vi "UI_FocusList.vi"() -> ()   [LabVIEW 2016]
uses:
  <vilib>/Utility/error.llb/DialogType.ctl
  DAQ-Display/PanelSplitToolkit/QueueManager.llb/Insert.vi
  DAQ-Display/PanelSplitToolkit/QueueManager.llb/Remove.vi
  Controls/DAQListOperation.ctl
  DAQ-Display/PanelSplitToolkit/QueueManager.llb/Valid?.vi
  DAQ-Display/PanelSplitToolkit/QueueManager.llb/Destroy.vi
  DAQ-Display/PanelSplitToolkit/QueueManager.llb/CreatQueue.vi
panel:
  out "波形图表":waveform(dbl)[](graph)
  out "ItemTag":string
  in  "Caller":string
  out "DAQList":i32(listbox)
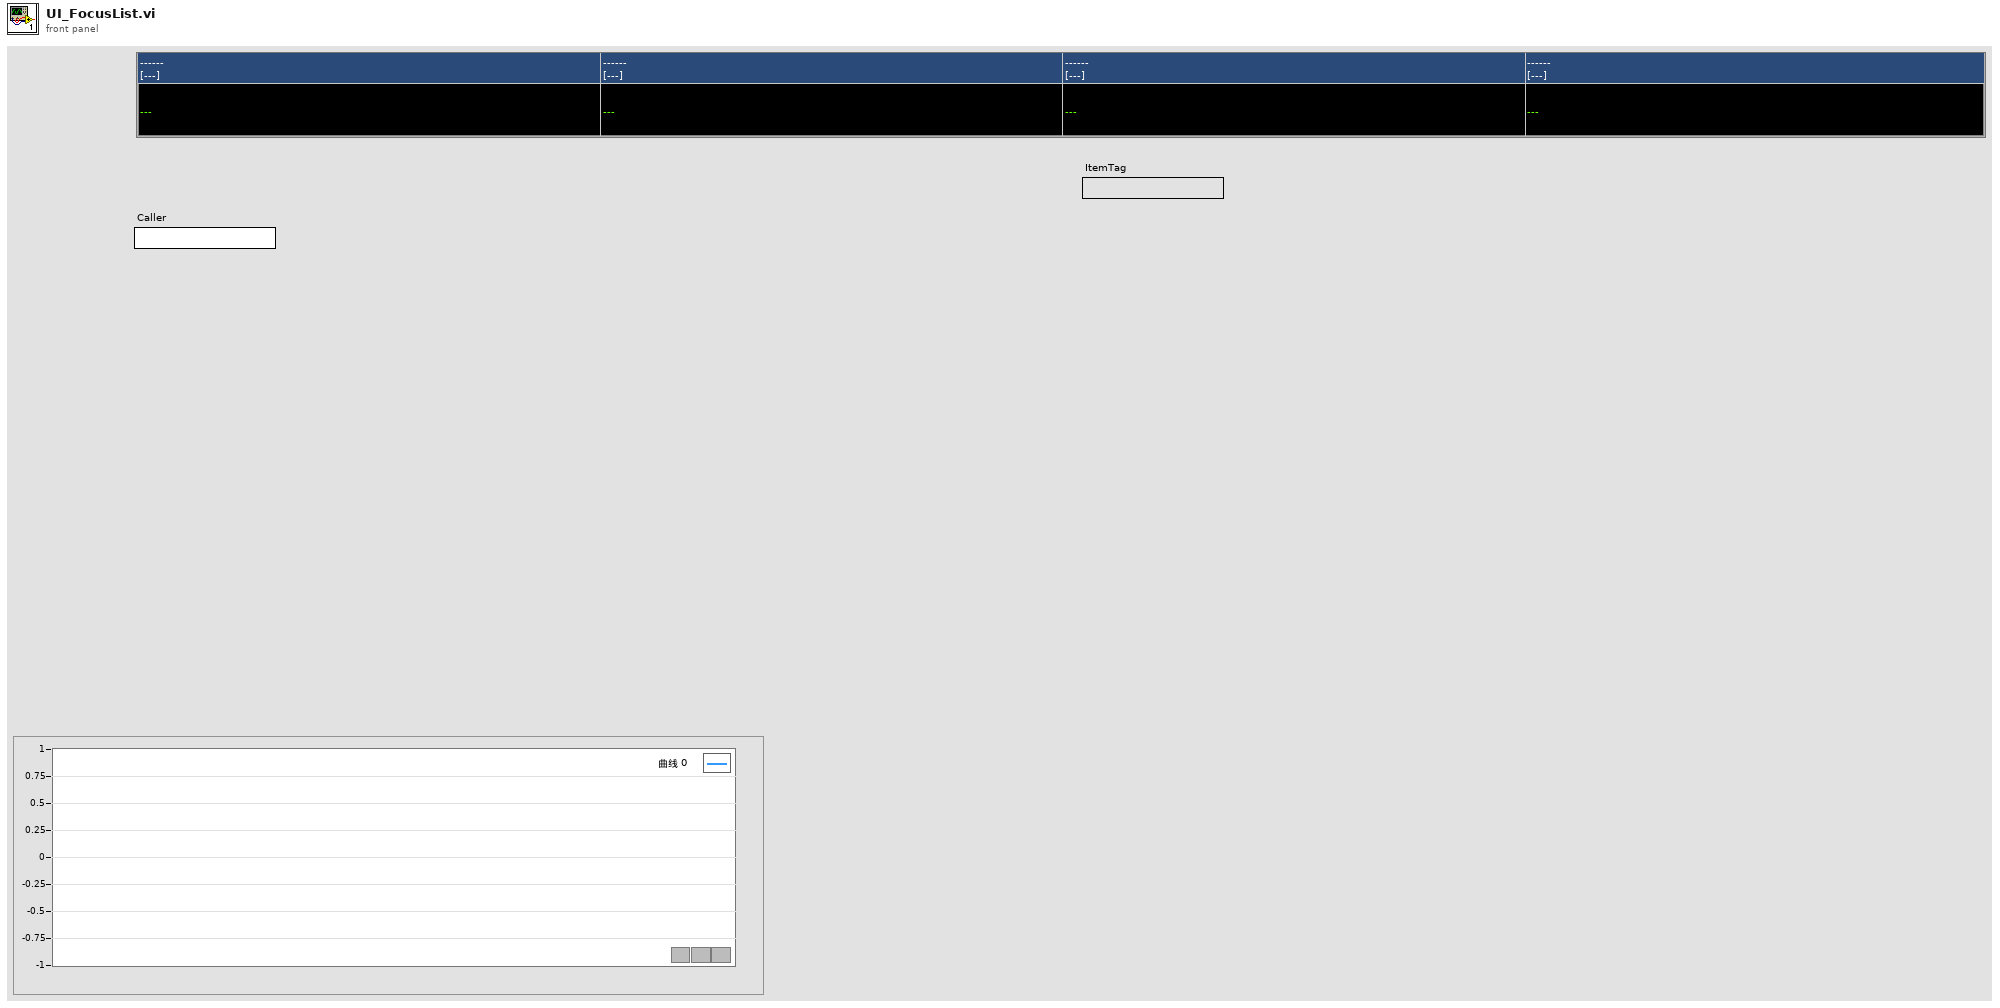
[diagram p1: front panel]
types:
  T1 = cluster{"error":errorcluster, "LocalQ":cluster{"LQName":string, "LQEvent":string, "LQData":variant}, "HighQ":cluster{"HQName":string, "HQEvent":string, "HQData":variant}}
  T2 = typedef "LVPoint32TypeDef.ctl" = cluster{"Horizontal":i32, "Vertical":i32}
  T3 = typedef "LVRowAndColumnTypeDef.ctl" = cluster{"Row":i32, "Column":i32}
  T4 = typedef "DAQListOperation.ctl" = enum16{"Init", "Clear", "Update Data", "Update CH Name", "Set List Property", "Get CHTag[]"}
  T5 = typedef "DialogType.ctl" = u16
  T6 = typedef "PCM PanelSplit.lvclass/Display Config.ctl" = cluster{"Display Mode":T7, "ChTag[]":string[], "window":T8, "Range":T9}
  T7 = typedef "PCM PanelSplit.lvclass/Display Mode.ctl" = enum16{"时域", "频谱", "功率谱"}
  T8 = typedef "NI_AALPro.lvlib/windowTd.ctl" = u32
  T9 = typedef "LVRangeTypeDef.ctl" = cluster{"Minimum":dbl, "Maximum":dbl, "Increment":dbl, "Minor Increment":dbl, "Start":dbl}
  T10 = cluster{"error":errorcluster, "LocalQ":cluster{"LQName":string, "LQEvent":string, "LQData":variant}, "HighQ":cluster{"HQName":string, "HQEvent":string, "HQData":variant}, "Display Config":T6, "波形图":refnum<vi>}
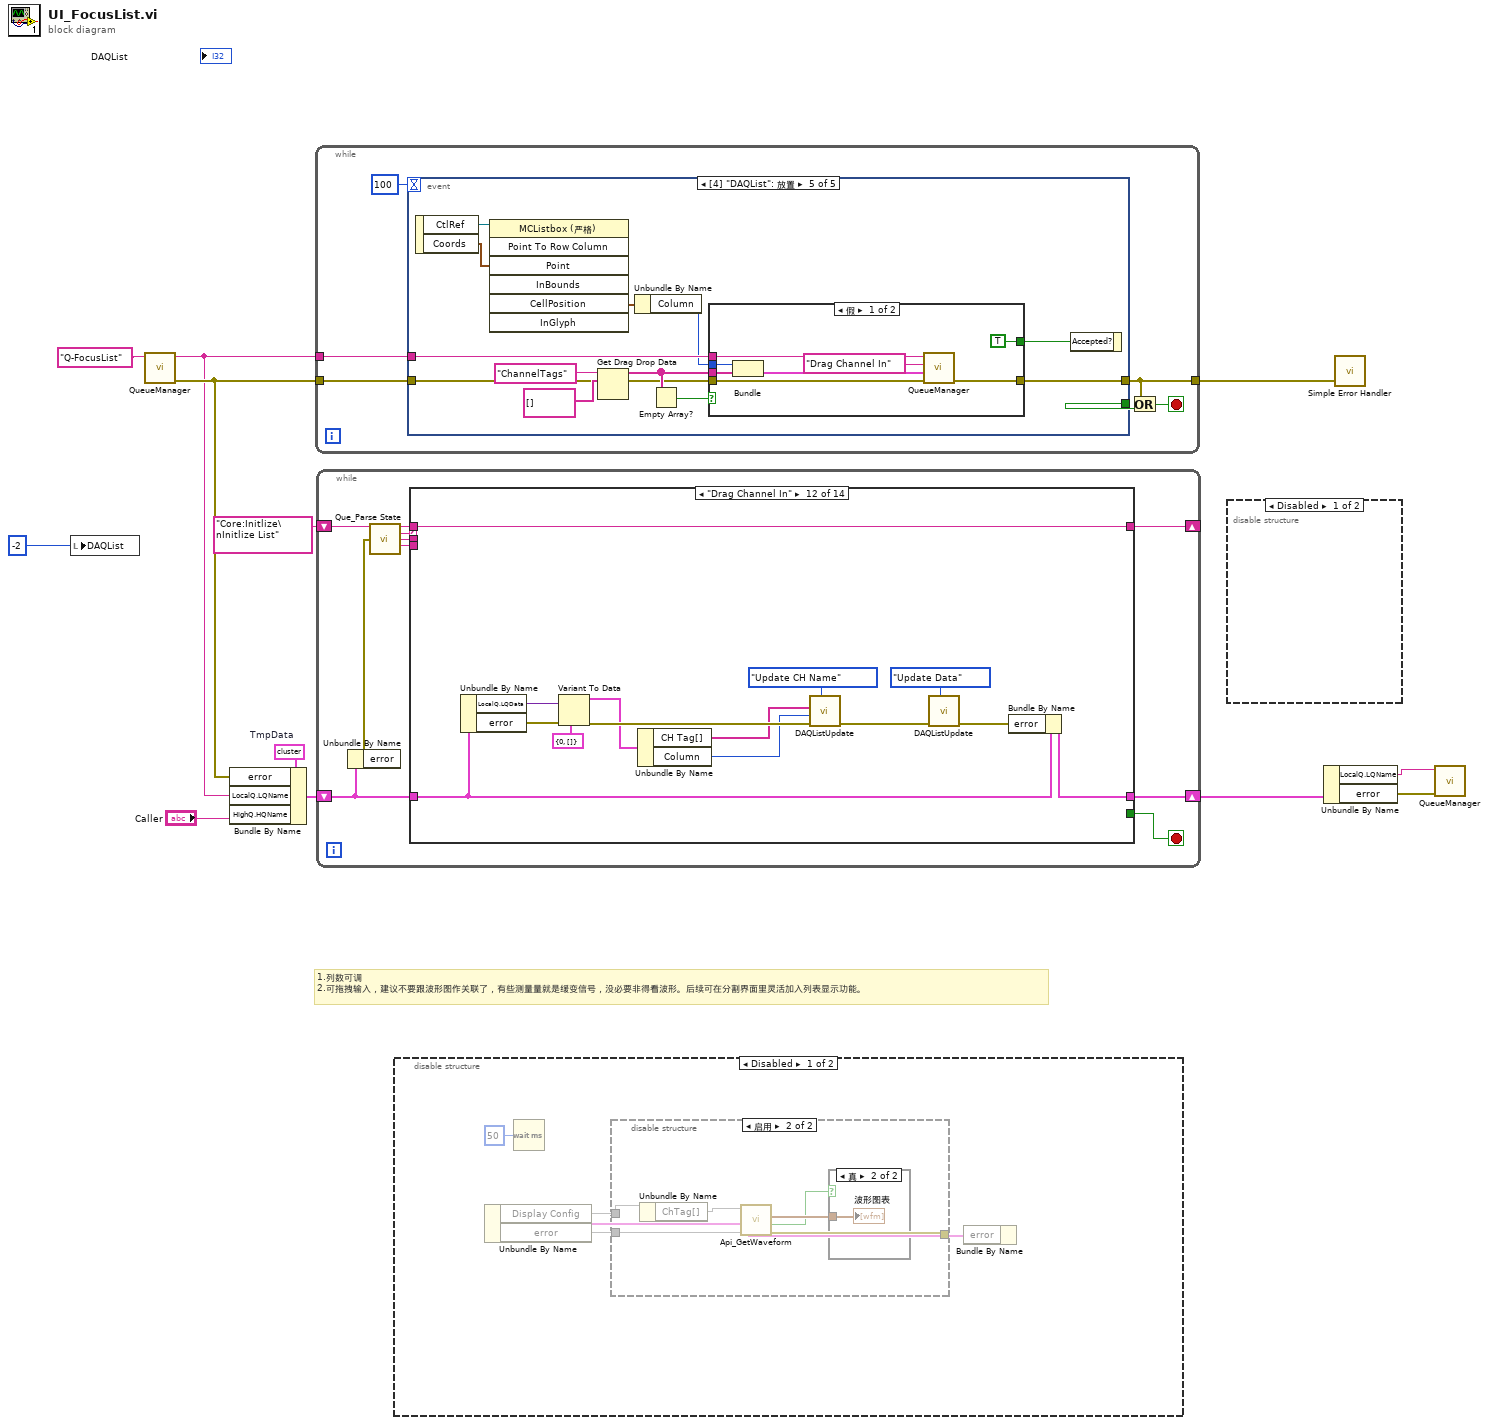
[diagram p0: block diagram]
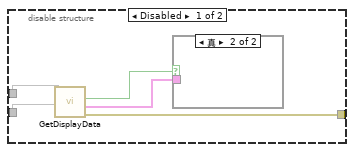
[diagram p2: hidden frame]
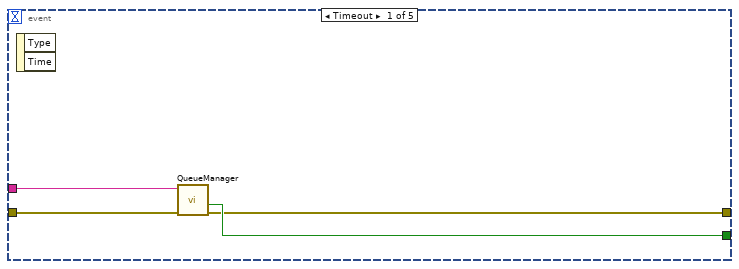
[diagram p7: hidden frame]
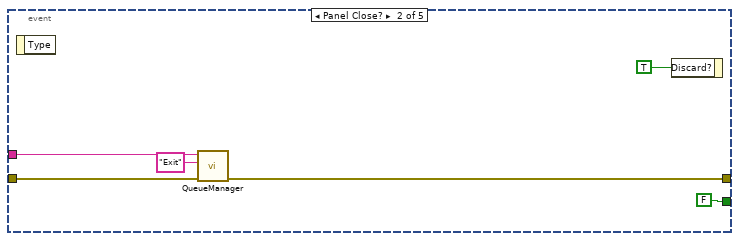
[diagram p8: hidden frame]
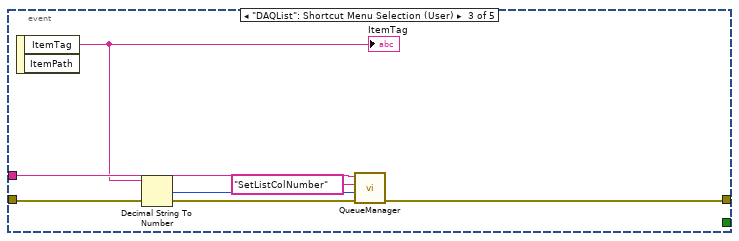
[diagram p9: hidden frame]
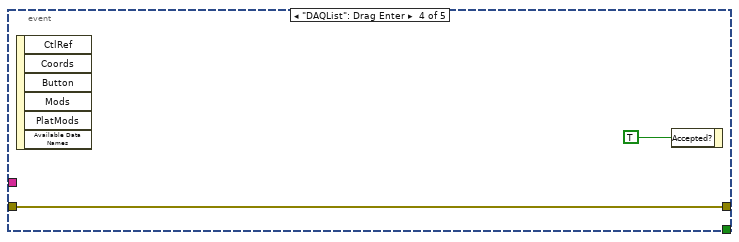
[diagram p10: hidden frame]
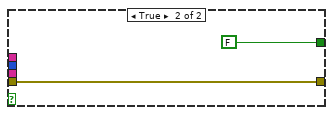
[diagram p11: hidden frame]
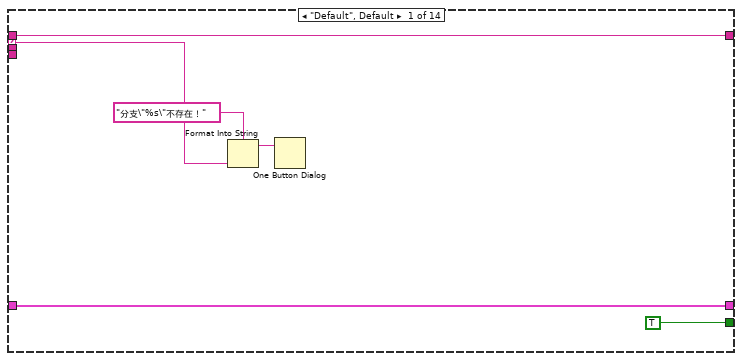
[diagram p12: hidden frame]
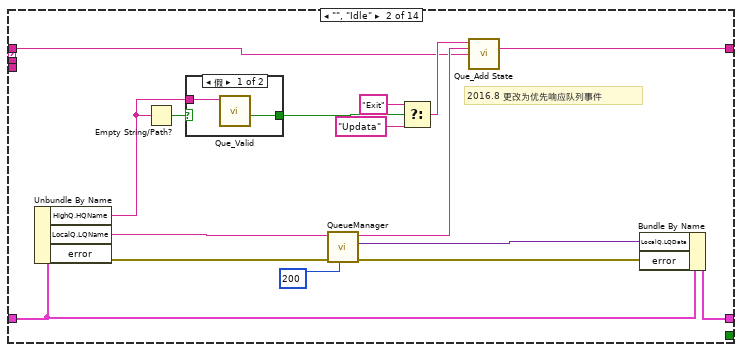
[diagram p13: hidden frame]
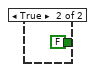
[diagram p14: hidden frame]
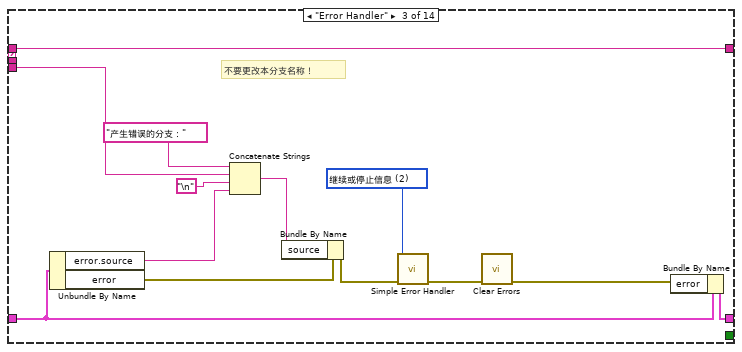
[diagram p15: hidden frame]
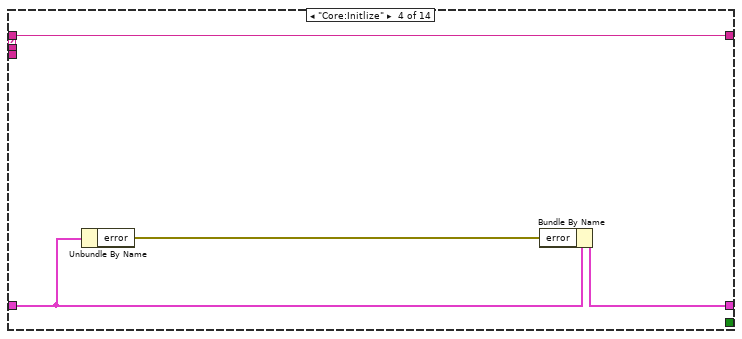
[diagram p16: hidden frame]
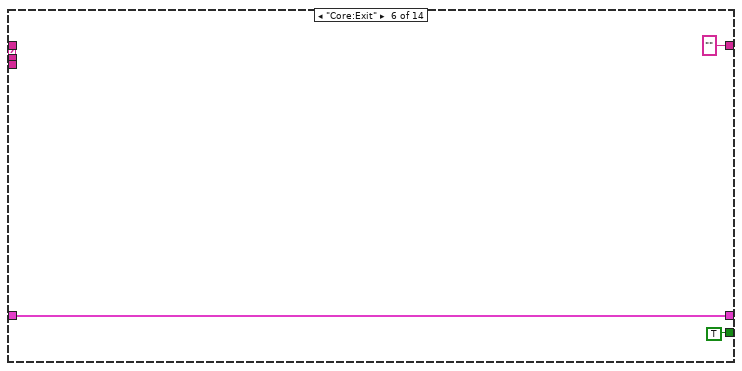
[diagram p18: hidden frame]
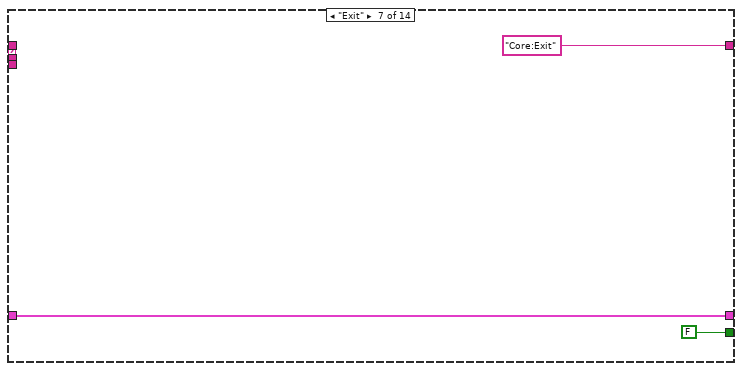
[diagram p19: hidden frame]
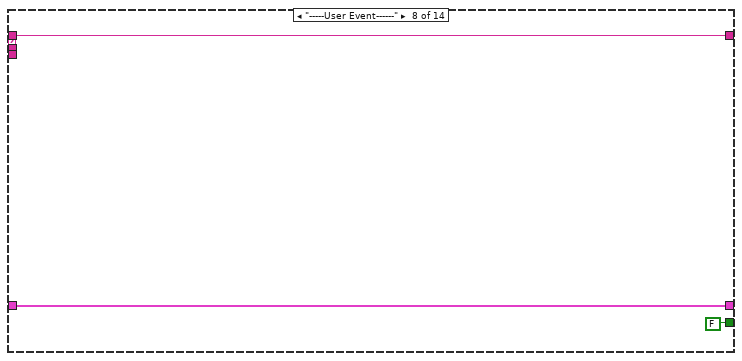
[diagram p20: hidden frame]
diagram:
  w8 = T1 {"error"={"status"=FALSE, "code"=0, "source"=""}, "LocalQ"={"LQName"="", "LQEvent"="", "LQData"=variant}, "HighQ"={"HQName"="", "HQEvent"="", "HQData"=variant}}  # TmpData
  # "1.列数可调\n2.可拖拽输入，建议不要跟波形图作关联了，有些测量量就是缓变信号，没必要非得看波形。后续可在分割界面里灵活加入列表显示功能。"
  n1 = local write "DAQList"(-2 ("Multicolumn Listbox")) -> ()
  n2 = call-poly "QueueManager.vi"("QueueName"="Q-FocusList") -> ("error out"=w4:errorcluster, "QueueName out"=w1:string)  [unwired: 9 in]
  n3 = Bundle By Name(cluster=w8, "error"=w4, "LocalQ.LQName"=w1, "HighQ.HQName"="Caller") -> (w7:T1)
  n4 = while {
    tunnel: w4 -> [w17]
    tunnel: w1 -> [w18]
    tunnel: [w14] -> w9
    stop <- w15 stop-if-true
    n5 = event shown="[4] \"DAQList\": 放置" {
      selector: _ -> [_ _ _ _ _]
      dyn-events: _ -> [_ _ _ _ _]
      timeout: 100 -> [_ _ _ _ _]
      tunnel: [w20 FALSE _ _ _] -> w16
      tunnel: w18 -> [w22 w27 w31 _ w43]
      tunnel: w17 -> [w21 w26 w33 w35 w44]
      tunnel: [w19 w25 w32 w35 w42] -> w14
      event Timeout {
        n6 = event-data() -> ()  [unwired: 1 in, 2 out]
        n7 = call-poly "QueueManager.vi"("error in (no error)"=w21, "Queue Name(unamed)"=w22) -> ("error out"=w19:errorcluster, "Not Exist?"=w20:bool)  [unwired: 8 in]
      }
      event Panel Close? {
        n8 = event-data() -> ()  [unwired: 1 in, 1 out]
        n9 = call-poly "QueueManager.vi"("error in"=w26, "Event"="Exit", "QueueName"=w27) -> ("error out"=w25:errorcluster)  [unwired: 7 in, 1 out]
        n10 = event-data("Discard?"=TRUE ("放弃？")) -> ()  [unwired: 1 in, 1 out]
      }
      event "DAQList": Shortcut Menu Selection (User) {
        n11 = event-data() -> ("ItemTag"=w30:string)  [unwired: 1 in, 1 out]
        "ItemTag" <- w30
        n12 = Decimal String To Number(string=w30) -> (number=w29:i32)  [unwired: 2 in, 1 out]
        n13 = call-poly "QueueManager.vi"("error in"=w33, "Data"=w29, "Event"="SetListColNumber", "QueueName"=w31) -> ("error out"=w32:errorcluster)  [unwired: 6 in, 1 out]
      }
      event "DAQList": Drag Enter {
        n14 = event-data() -> ()  [unwired: 1 in, 6 out]
        n15 = event-data("Accepted?"=TRUE) -> ()  [unwired: 1 in, 1 out]
      }
      event "DAQList": Drop {
        n16 = event-data() -> ("CtlRef"=w40:refnum<vi>, "Coords"=w39:T2)  [unwired: 1 in]
        n17 = invoke class="MCListbox (严格)" method="Point To Row Column"(reference=w40, "Point"=w39) -> ("CellPosition"=w38:T3)  [unwired: 5 in, 6 out]
        n18 = Get Drag Drop Data(8:string[] [], 9:"ChannelTags" ("数据名称")) -> (3:w47:string[])  [unwired: 1 in, 1 out]
        n19 = Unbundle By Name(w38) -> ("Column"=w37:i32)
        n20 = Empty Array?(array=w47) -> (empty?=w48:bool)
        n21 = case shown="假" w48 {
          tunnel: w44 -> [w56 w58]
          tunnel: [w55 w58] -> w42
          tunnel: w43 -> [w54 _]
          tunnel: w47 -> [w50 _]
          tunnel: [TRUE ("放弃？") FALSE ("放弃？")] -> w41
          tunnel: w37 -> [w51 _]
          frame False {
            n22 = Bundle("Column"=w51, w50) -> (w49:cluster{"Column":i32, string[]})  [unwired: 1 in]
            n23 = call-poly "QueueManager.vi"("error in"=w56, "Data"=w49, "Event"="Drag Channel In", "QueueName"=w54) -> ("error out"=w55:errorcluster)  [unwired: 6 in, 1 out]
          }
          frame True {
          }
        }
        n24 = event-data("Accepted?"=w41) -> ()  [unwired: 1 in, 1 out]
      }
    }
    n25 = Or(x=w14, y=w16) -> (x .or. y?=w15:bool)
  }
  n26 = while {
    shift-right: [w62] -> w10
    shift-left: w7 -> [w63]
    shift-right: [w61] -> _
    shift-left: "Core:Initlize\nInitlize List" -> [w68]
    stop <- w65 stop-if-true
    n27 = Unbundle By Name(w63) -> ("error"=w64:errorcluster)
    n28 = call "Que_Parse State.vi"("State Queue"=w68, "Error In (no error)"=w64) -> ("Remaining States"=w67:string, "Current State"=w66:string, "Arguments"=w60:string, "PreState"=w59:string)  [unwired: 10 in]
    n29 = case shown="\"Drag Channel In\"" w66 {
      selector: w66 -> [w72 _ _ _ _ _ _ _ _ _ _ _ _ _]
      tunnel: w67 -> [w73 w75 w106 w110 w112 _ _ w119 w128 w136 w150 w164 w178 w184]
      tunnel: w60 -> [_ _ _ _ _ _ _ _ _ _ _ _ _ _]
      tunnel: [TRUE _ _ _ _ TRUE FALSE FALSE _ _ _ _ _ _] -> w65
      tunnel: w63 -> [w74 w85 w103 w108 w111 w114 w117 w120 w124 w131 w149 w163 w177 w183]
      tunnel: [w74 w89 w102 w109 w111 w114 w117 w120 w122 w130 w143 w162 w176 w182] -> w62
      tunnel: [w73 w87 w106 w110 w112 "" ("Remaining States") "Core:Exit" ("Remaining States") w119 w128 w135 w150 w164 w178 w184] -> w61
      tunnel: w59 -> [_ _ w100 _ _ _ _ _ _ _ _ _ _ _]
      frame "Default", Default {
        n30 = Format Into String(format string="分支\"%s\"不存在！" ("格式字符串"), w72) -> (resulting string=w71:string)  [unwired: 2 in, 1 out]
        n31 = One Button Dialog(message=w71) -> ()  [unwired: 1 in, 1 out]
      }
      frame "", "Idle" {
        # "2016.8 更改为优先响应队列事件"
        n32 = Unbundle By Name(w85) -> ("HighQ.HQName"=w79:string, "LocalQ.LQName"=w84:string, "error"=w83:errorcluster)
        n33 = Empty String/Path?(string/path=w79) -> (empty?=w82:bool)
        n34 = case shown="假" w82 {
          tunnel: [w92 FALSE ("Not Exist?")] -> w81
          tunnel: w79 -> [w91 _]
          frame False {
            n35 = call "Que_Valid.vi"("Queue Name(unamed)"=w91) -> ("Not Exist?"=w92:bool)  [unwired: 9 in, 1 out]
          }
          frame True {
          }
        }
        n36 = call-poly "QueueManager.vi"("Time out(-1)"=200, "error in (no error)"=w83, "Queue Name"=w84) -> ("error out"=w90:errorcluster, "Data"=w88:variant, "Event"=w76:string)  [unwired: 5 in, 1 out]
        n37 = Select(t="Exit" ("Event"), s=w81, f="Updata") -> (s? t:f=w77:string)
        n38 = call "Que_Add State.vi"("State(s) in Front (\"\")"=w77, "State(s) in (\"\")"=w76, "State(s) at Back (\"\")"=w75) -> ("States Out"=w87:string)  [unwired: 12 in]
        n39 = Bundle By Name(cluster=w85, "LocalQ.LQData"=w88, "error"=w90) -> (w89:T1)
      }
      frame "Error Handler" {
        w101 = T5 2 items=["无对话框", "确定信息", "继续或停止信息", "确定信息＋警告", "继续/停止+警告"] ("type of dialog (OK msg:1)")
        # "不要更改本分支名称！"
        n40 = Unbundle By Name(w103) -> ("error.source"=w94:string, "error"=w96:errorcluster)
        n41 = Concatenate Strings("产生错误的分支：" ("字符串"), w100, "\n", w94) -> (w97:string)
        n42 = Bundle By Name(cluster=w96, "source"=w97) -> (w95:errorcluster)
        n43 = call <vilib>:"Simple Error Handler.vi"("type of dialog (OK msg:1)"=w101, "error in (no error)"=w95) -> ("error out"=w104:errorcluster)  [unwired: 3 in, 4 out]
        n44 = call <vilib>:"Clear Errors.vi"("error in (no error)"=w104) -> ("error out"=w105:errorcluster)  [unwired: 5 in, 1 out]
        n45 = Bundle By Name(cluster=w103, "error"=w105) -> (w102:T1)
      }
      frame "Core:Initlize" {
        n46 = Unbundle By Name(w108) -> ("error"=w107:errorcluster)
        n47 = Bundle By Name(cluster=w108, "error"=w107) -> (w109:T1)
      }
      frame "Core:DataInitlize" {
      }
      frame "Core:Exit" {
      }
      frame "Exit" {
      }
      frame "-----User Event------" {
      }
      frame "Initlize List" {
        # "主线程会在本VI插入subpannel时发送一次命令，以匹配主VI大小"
        n48 = Unbundle By Name(w124) -> ("error"=w125:errorcluster)
        n49 = control-ref of="DAQList"() -> (w127:refnum<vi>)
        n50 = call "DAQListUpdate.vi"("Comm"=DAQListOperation."Init", "error in (no error)"=w125, "List* in"=w127) -> ("error out"=w123:errorcluster)  [unwired: 6 in, 2 out]
        n51 = Bundle By Name(cluster=w124, "error"=w123) -> (w122:T1)
      }
      frame "Updata" {
        # "更新数据"
        n52 = Wait (ms)(milliseconds to wait=u32 100 ("等待时间（毫秒）")) -> ()  [unwired: 1 out]
        n53 = Unbundle By Name(w131) -> ("error"=w129:errorcluster)
        n54 = call "DAQListUpdate.vi"("Comm"=DAQListOperation."Update Data", "error in (no error)"=w129) -> ("error out"=w133:errorcluster)  [unwired: 7 in, 2 out]
        n55 = disable-structure shown="启用" {
          disable-tunnel: w136 -> [w139 w140]
          disable-tunnel: [w138 w140] -> w135
          frame Disabled {
            n56 = call "Que_Add State.vi"("State(s) in (\"\")"=w139, "State(s) at Back (\"\")"="Idle\nUpdata" ("State(s) at Back (\"\")")) -> ("States Out"=w138:string)  [unwired: 13 in]
          }
          frame Enabled {
          }
        }
        n57 = Bundle By Name(cluster=w131, "error"=w133) -> (w130:T1)
      }
      frame "SetListColNumber" {
        n58 = Unbundle By Name(w149) -> ("LocalQ.LQData"=w146:variant, "error"=w148:errorcluster)
        n59 = Variant To Data(error in=w148, type=0 ("ColNumbers"), Variant=w146) -> (data=w144:i32, error out=w147:errorcluster)
        n60 = call "DAQListUpdate.vi"("Comm"=DAQListOperation."Set List Property", "error in (no error)"=w147, "ColNumbers"=w144) -> ("error out"=w142:errorcluster)  [unwired: 6 in, 2 out]
        n61 = Bundle By Name(cluster=w149, "error"=w142) -> (w143:T1)
      }
      frame "Drag Channel In" {
        n62 = Unbundle By Name(w163) -> ("LocalQ.LQData"=w160:variant, "error"=w161:errorcluster)
        n63 = Variant To Data(error in=w161, type=cluster{"Column":i32, "CH Tag[]":string[]} {"Column"=0, "CH Tag[]"=[]} ("输出簇"), Variant=w160) -> (data=w157:cluster{"Column":i32, "CH Tag[]":string[]}, error out=w158:errorcluster)
        n64 = Unbundle By Name(w157) -> ("CH Tag[]"=w155:string[], "Column"=w156:i32)
        n65 = call "DAQListUpdate.vi"("Comm"=DAQListOperation."Update CH Name", "error in (no error)"=w158, "ColNumbers"=w156, "Channels info"=w155) -> ("error out"=w153:errorcluster)  [unwired: 5 in, 2 out]
        n66 = call "DAQListUpdate.vi"("Comm"=DAQListOperation."Update Data", "error in (no error)"=w153) -> ("error out"=w152:errorcluster)  [unwired: 7 in, 2 out]
        n67 = Bundle By Name(cluster=w163, "error"=w152) -> (w162:T1)
      }
      frame "COM : Load" {
        # "从文件中载入存储信息"
        n68 = Unbundle By Name(w177) -> ("LocalQ.LQData"=w174:variant, "error"=w175:errorcluster)
        n69 = Variant To Data(error in=w175, type=string[] [], Variant=w174) -> (data=w167:string[], error out=w172:errorcluster)
        n70 = Array Size(array=w167) -> (size(s)=w166:i32)
        n71 = call "DAQListUpdate.vi"("Comm"=DAQListOperation."Set List Property", "error in (no error)"=w172, "ColNumbers"=w166) -> ("error out"=w171:errorcluster)  [unwired: 6 in, 2 out]
        n72 = call "DAQListUpdate.vi"("Comm"=DAQListOperation."Update CH Name", "error in (no error)"=w171, "ColNumbers"=0, "Channels info"=w167) -> ("error out"=w170:errorcluster)  [unwired: 5 in, 2 out]
        n73 = Bundle By Name(cluster=w177, "error"=w170) -> (w176:T1)
      }
      frame "COM : Save" {
        # "不需要此分支，直接用这个功能全局获取CHTag[]存入文件即可"
        n74 = Unbundle By Name(w183) -> ("error"=w179:errorcluster)  [unwired: 1 out]
        n75 = call "DAQListUpdate.vi"("Comm"=DAQListOperation."Get CHTag[]", "error in (no error)"=w179) -> ("error out"=w181:errorcluster)  [unwired: 7 in, 2 out]
        n76 = Bundle By Name(cluster=w183, "error"=w181) -> (w182:T1)
      }
    }
  }
  n77 = disable-structure shown="Disabled" {
    frame Disabled {
      n78 = Unbundle By Name() -> (w188:T10, "Display Config"=w190, "error"=w189)
      n79 = Wait (ms)(milliseconds to wait=u32 50 ("等待时间（毫秒）")) -> ()  [unwired: 1 out]
      n80 = disable-structure shown="启用" {
        disable-tunnel: w190 -> [w195 w201]
        disable-tunnel: w189 -> [w194 w199]
        disable-tunnel: [w191 w198] -> w187
        frame Disabled {
          n81 = call "GetDisplayData.vi"("error in"=w194, "Display Config"=w195) -> ("error out"=w191:errorcluster, "Data"=w193:cluster{"f0":dbl, "df":dbl, "magnitude":dbl[]}[], "Valid?"=w192:bool)  [unwired: 7 in]
          n82 = case shown="真" w192 {
            tunnel: w193 -> [_ _]
            frame False {
            }
            frame True {
            }
          }
        }
        frame Enabled {
          n83 = Unbundle By Name(w201) -> ("ChTag[]"=w200)
          n84 = call "Api_GetWaveform.vi"("error in (no error)"=w199, "Tags[]"=w200) -> ("error out"=w198:errorcluster, "Display?"=w196:bool, "Wave[]"=w197:waveform(dbl)[])  [unwired: 7 in]
          n85 = case shown="真" w196 {
            tunnel: w197 -> [_ w202]
            frame False {
            }
            frame True {
              "波形图表" <- w202
            }
          }
        }
      }
      n86 = Bundle By Name(cluster=w188, "error"=w187) -> (w186:cluster{})
    }
    frame Enabled {
    }
  }
  n87 = disable-structure shown="Disabled" {
    frame Disabled {
    }
    frame Enabled {
    }
  }
  n88 = Unbundle By Name(w10) -> ("LocalQ.LQName"=w5:string, "error"=w11:errorcluster)
  n89 = call <vilib>:"Simple Error Handler.vi"("error in (no error)"=w9) -> ()  [unwired: 4 in, 5 out]
  n90 = call-poly "QueueManager.vi"("error in (no error)"=w11, "QueeuName"=w5) -> ()  [unwired: 9 in, 1 out]
